vi "Unflatten Socket CAN Header.vi"(8 "error in (no error)":errorcluster, 10 "Bytes in":u8[](array[numeric]), 11 "pcap Parse and Build in":refnum<class "pcap_Parse_Build_CIF.lvclass">) -> (0 "error out":errorcluster, 1 "Socket CAN Header":T1 {"CANID and Flags" format="%.0x"; "FD Flags" format="%.0x"}, 2 "Bytes out":u8[](array[numeric]), 3 "pcap Parse and Build out":refnum<class "pcap_Parse_Build_CIF.lvclass">)   [LabVIEW 2021, in "pcap_Parse_Build_CIF.lvclass"]
uses:
  pcap_Parse_Build_CIF.lvclass
  Typedef/Format Specific/Socket CAN Header.ctl
  pcap_Parse_Build_CIF.lvclass/pcap_Parse_Build_CIF.ctl
  Typedef/Errors.ctl
  <vilib>/CIF Foundation/CIF Utilities/DataTypes/Typedef/Endian.ctl
  <vilib>/CIF Foundation/CIF Utilities/Errors/Append Error Location.vi
  <vilib>/CIF Foundation/CIF Utilities/DataTypes/DataTypes_CIF_U.lvlib
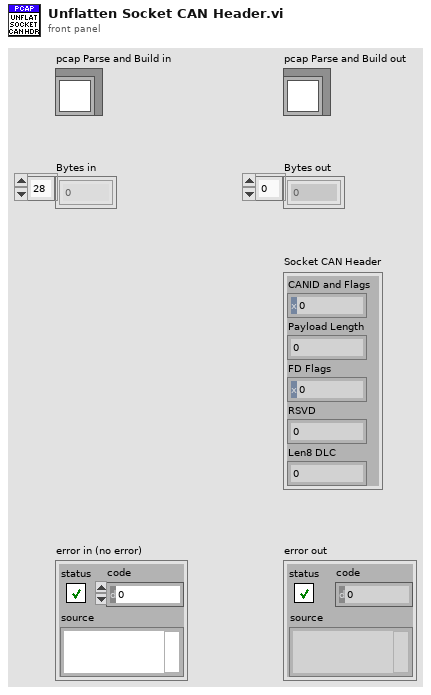
[diagram p1: front panel]
types:
  T1 = typedef "pcap_Parse_Build_CIF.lvclass/Socket CAN Header.ctl" = cluster{"CANID and Flags":u32, "Payload Length":u8, "FD Flags":u8, "RSVD":u8, "Len8 DLC":u8}
  T2 = typedef "pcap_Parse_Build_CIF.lvclass/Errors.ctl" = enum16{"Invalid Global Header", "Out of Data"}
  T3 = typedef "DataTypes_CIF_U.lvlib/Endian.ctl" = enum16{"Little Endian", "Big Endian"}
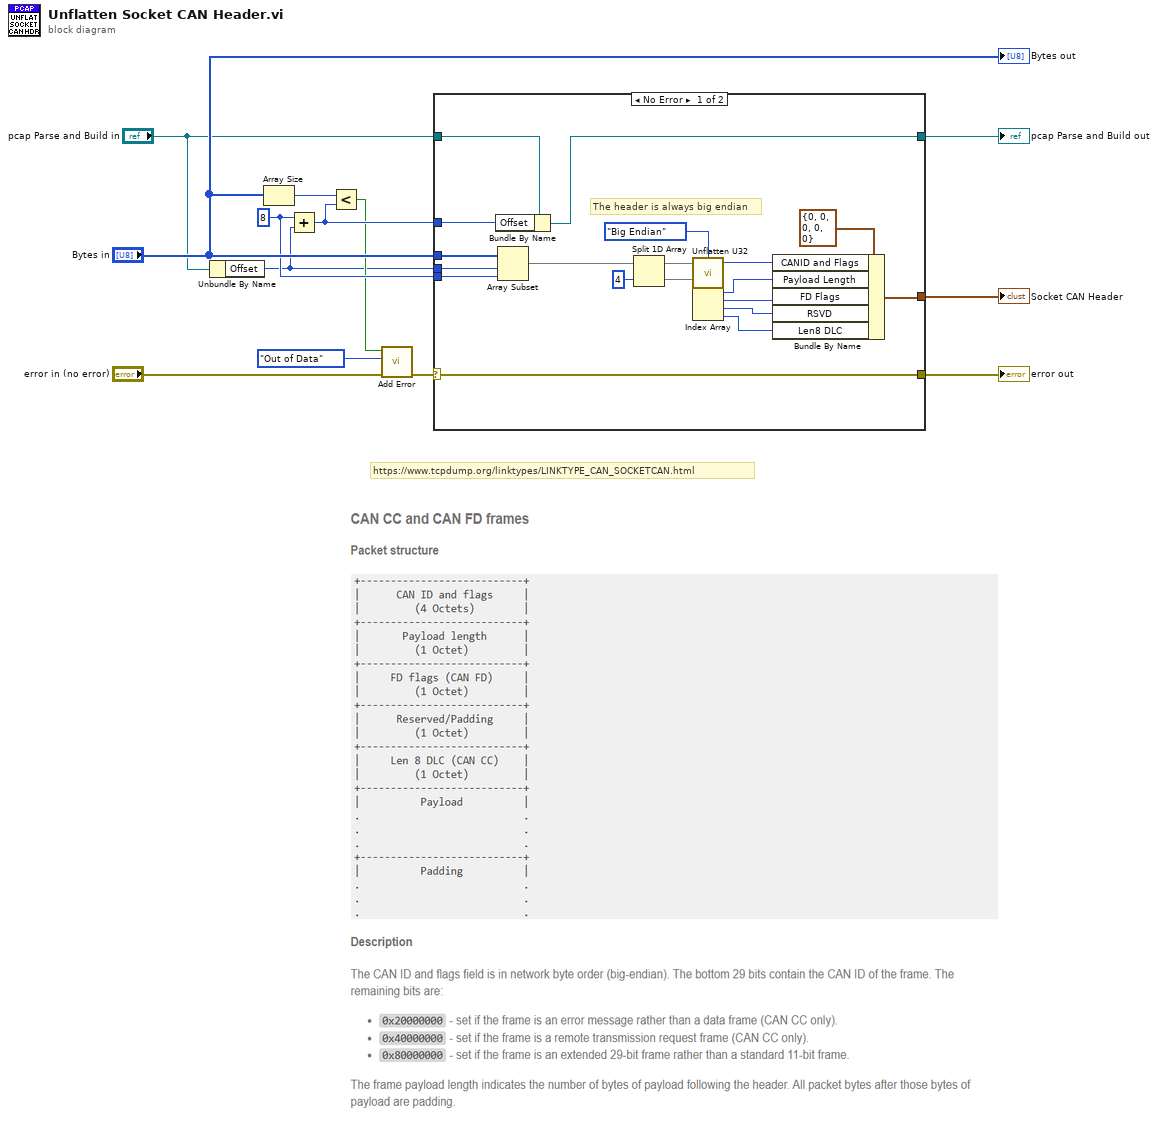
[diagram p0: block diagram]
diagram:
  w11 = 8 ("length")
  # "https://www.tcpdump.org/linktypes/LINKTYPE_CAN_SOCKETCAN.html"
  n1 = Unbundle By Name("pcap Parse and Build in") -> ("Offset"=w4:i32)
  n2 = Array Size(array="Bytes in") -> (size(s)=w6:i32)
  n3 = Add(x=w11, y=w4) -> (x+y=w12:i32)
  n4 = Less?(x=w6, y=w12) -> (x < y?=w10:bool)
  n5 = call "Add Error.vi"("error in (no error)"="error in (no error)", "Error"=Errors."Out of Data", "Insert Error"=w10) -> ("error out"=w7:errorcluster)  [unwired: 8 in]
  n6 = case shown="No Error" w7 {
    selector: w7 -> [w20 w34]
    tunnel: [w20 w34] -> w5
    tunnel: "Bytes in" -> [w32 _]
    tunnel: w12 -> [w28 _]
    tunnel: w11 -> [w31 _]
    tunnel: w4 -> [w30 _]
    tunnel: "pcap Parse and Build in" -> [w29 w33]
    tunnel: [w26 w33] -> w2
    tunnel: [w18 _] -> w1
    frame No Error {
      # "The header is always big endian"
      n7 = Bundle By Name(cluster=w29, "Offset"=w28) -> (w26:refnum<class "pcap_Parse_Build_CIF.lvclass">)
      n8 = Array Subset(array=w32, index=w30, length=w31) -> (w27:u8[])
      n9 = Split 1D Array(array=w27, index=4) -> (first subarray=w23:u8[], second subarray=w21:u8[])
      n10 = call <vilib>:"Unflatten U32.vi"("Flat Data"=w23, "Endian"=Endian."Big Endian") -> ("U32"=w19:u32)  [unwired: 3 in]
      n11 = Index Array(array=w21) -> (element #1=w17:u8, element #2=w16:u8, element #3=w15:u8, element #4=w14:u8)  [unwired: 4 in]
      n12 = Bundle By Name(cluster=T1 {"CANID and Flags"=0, "Payload Length"=0, "FD Flags"=0, "RSVD"=0, "Len8 DLC"=0} ("SocketCAN Header"), "CANID and Flags"=w19, "Payload Length"=w17, "FD Flags"=w16, "RSVD"=w15, "Len8 DLC"=w14) -> (w18:T1)
    }
    frame Error {
    }
  }
  "pcap Parse and Build out" <- w2
  "error out" <- w5
  "Socket CAN Header" <- w1
  "Bytes out" <- "Bytes in"
